vi "ClearBuffer.vi"(7 "SMU":T1, 8 "Error In":errorcluster, 10 "Buffer":u8=1 min=1 max=2 step=1, 11 "Keithley 2602 In":refnum<visa-resource-name>) -> (0 "Error Out":errorcluster, 3 "Keithley 2602 Out":refnum<visa-resource-name>)   [LabVIEW 2013, in "Keithley-2602.lvlib"]
uses:
  Keithley-2602.lvlib
  Controls/SMU.ctl
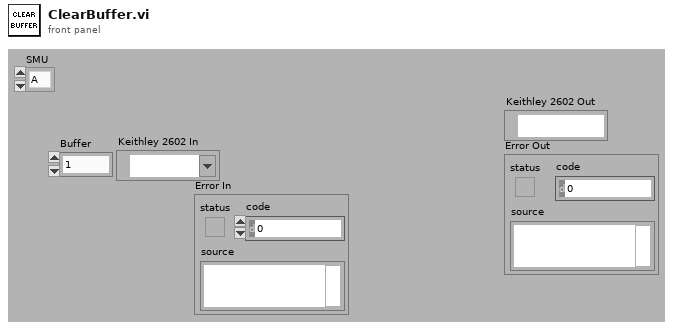
[diagram p1: front panel]
types:
  T1 = typedef "Keithley-2602.lvlib/SMU.ctl" = enum16{"A", "B"}
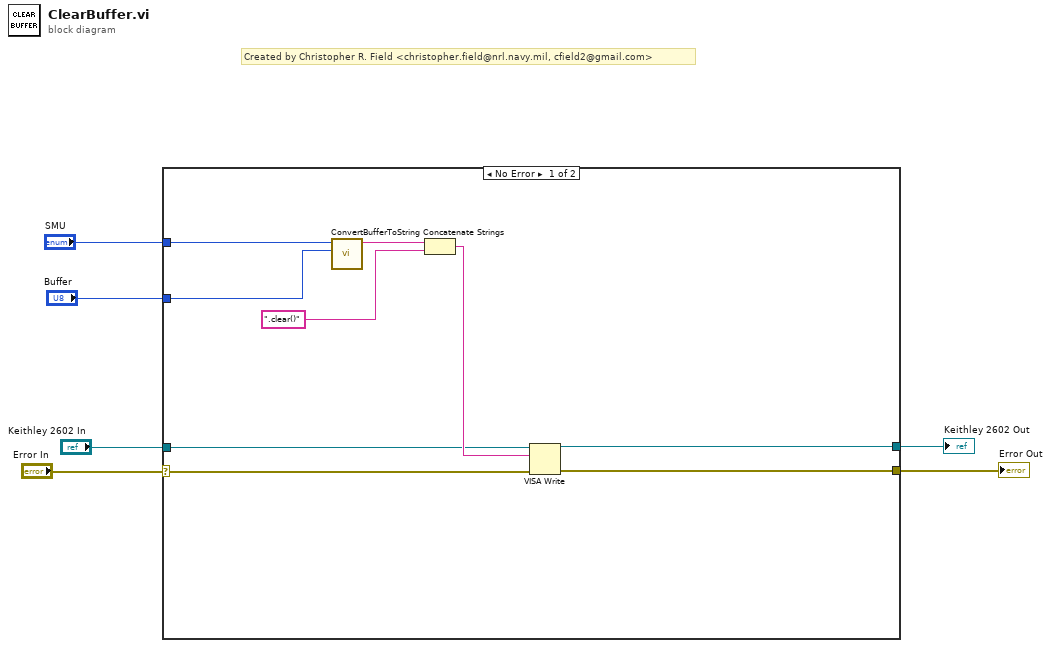
[diagram p0: block diagram]
diagram:
  # "Created by Christopher R. Field <christopher.field@nrl.navy.mil, cfield2@gmail.com>"
  n1 = case shown="No Error" "Error In" {
    selector: "Error In" -> [w7 w16]
    tunnel: "Buffer" -> [w15 _]
    tunnel: "Keithley 2602 In" -> [w11 w17]
    tunnel: [w10 w17] -> w4
    tunnel: [w9 w16] -> w3
    tunnel: "SMU" -> [w8 _]
    frame No Error {
      n2 = call "ConvertBufferToString.vi"("Buffer"=w15, "SMU"=w8) -> ("Buffer"=w14:string)  [unwired: 9 in]
      n3 = Concatenate Strings(w14, ".clear()") -> (w12:string)
      n4 = VISA Write(VISA resource name=w11, write buffer=w12, error in (no error)=w7) -> (VISA resource name out=w10:refnum<visa-resource-name>, error out=w9:errorcluster)  [unwired: 1 out]
    }
    frame Error {
    }
  }
  "Keithley 2602 Out" <- w4
  "Error Out" <- w3
